vi "convertidor de pasos a distancia v1.vi"(9 "Set 0 vitual":bool, 10 "Respuesta Zaber":T7 {"Command" items=["Constant Speed Tracking"=8, "Echo"=55, "Error"=255, "Home"=1, "Limit Active"=9, "Manual Move Tracking"=10, "Move Absolute"=20, "Move at Constant Speed"=22, "Move Relative"=21, "Renumber"=2, "Restore Settings"=36, "Stop"=23]}, 11 "Datos adquisición Input":T1={"Equipo a Utilizar"=enum."TDS 2012B Osciloscope", "Montura"=enum."Motor Bipolar", "Datos Zaber"={"Sentido de Adquisición"=FALSE, "Comenzar Desde Home?"=FALSE, "Distancia a recorrer (um)"=0.0, "Pasos motor"=0, "Distancia entre Lecturas (um)"=0.0, "Puerto"=""}, "Datos Bipolar/Unipolar"={"Puerto COM"="", "Pasos entre Lecturas"=0, "Numero de lecturas"=0, "Sentido del motor"=TRUE}, "Datos Archivo"={"Ruta Archivo"=path "", "Nombre de Prueba"=""}, "Datos actuales"={"Montura"="", "Equipo"="", "Posición Actual"="", "Distancia Total a recorrer"="", "distancia Entre lecturas"="", "Pasos entre lecturas"=""}, "Datos a Guardar In"={"Datos Cursor Tektronix"="", "Datos Lokin"="", "Posición Cero"=0.0, "Posición Actual"=0.0}, "Datos Osciloscopio"={"Sesión Visa Osciloscopio"="Tektronix_TDS2012C", "Tipo de Adquisición"=enum."Voltaje Pico Pico", "Canal a Utilizar"=enum."Canal 1", "Parametros de Adquisición"=enum."Una Muestra", "Número Promedio"=2}, "Datos Lock In"={"Visa Lock in"="Tektronix_TDS2012C"}} {"Datos Osciloscopio"."Número Promedio" min=2 max=20; "Datos a Guardar In"."Posición Actual" format="%#_10f"; "Datos a Guardar In"."Posición Cero" format="%#_10f"; "Datos Bipolar/Unipolar"."Numero de lecturas" max=910098 step=1}) -> (1 "Respuesta conversión zaber":dbl[unit], 3 "Datos adquisición Out":T1={"Equipo a Utilizar"=enum."TDS 2012B Osciloscope", "Montura"=enum."Motor Bipolar", "Datos Zaber"={"Sentido de Adquisición"=FALSE, "Comenzar Desde Home?"=FALSE, "Distancia a recorrer (um)"=0.0, "Pasos motor"=0, "Distancia entre Lecturas (um)"=0.0, "Puerto"=""}, "Datos Bipolar/Unipolar"={"Puerto COM"="", "Pasos entre Lecturas"=0, "Numero de lecturas"=0, "Sentido del motor"=TRUE}, "Datos Archivo"={"Ruta Archivo"=path "", "Nombre de Prueba"=""}, "Datos actuales"={"Montura"="", "Equipo"="", "Posición Actual"="", "Distancia Total a recorrer"="", "distancia Entre lecturas"="", "Pasos entre lecturas"=""}, "Datos a Guardar In"={"Datos Cursor Tektronix"="", "Datos Lokin"="", "Posición Cero"=0.0, "Posición Actual"=0.0}, "Datos Osciloscopio"={"Sesión Visa Osciloscopio"="Tektronix_TDS2012C", "Tipo de Adquisición"=enum."Voltaje Pico Pico", "Canal a Utilizar"=enum."Canal 1", "Parametros de Adquisición"=enum."Una Muestra", "Número Promedio"=2}, "Datos Lock In"={"Visa Lock in"="Tektronix_TDS2012C"}} {"Datos Osciloscopio"."Número Promedio" min=2 max=20; "Datos a Guardar In"."Posición Actual" format="%#_10f"; "Datos a Guardar In"."Posición Cero" format="%#_10f"; "Datos Bipolar/Unipolar"."Numero de lecturas" max=910098 step=1}, 5 "Seguir Moviendo":bool)   [LabVIEW 2020]
doc: "Este Vi convierte el dato recibido de el driver zaber a distancia actual en unidades de distancia"
uses:
  <instrlib>/ZaberTSeries/Public/Utility/Response.ctl
  <instrlib>/ZaberTSeries/ZaberTSeries.lvlib
  Type Definitions/Asistente de adquisicion Cluster.ctl
  Type Definitions/Datos a Guardar.ctl
  Type Definitions/datos osciloscopio.ctl
  Type Definitions/Datos Zaber.ctl
  Type Definitions/parametros motores.ctl
  H:/Mi unidad/Departamento de Ingenieria/Investigadores/Gabriel Ramos/Proyecto Monturas v13/LV Source/Type Definitions/Tipos de montura.ctl
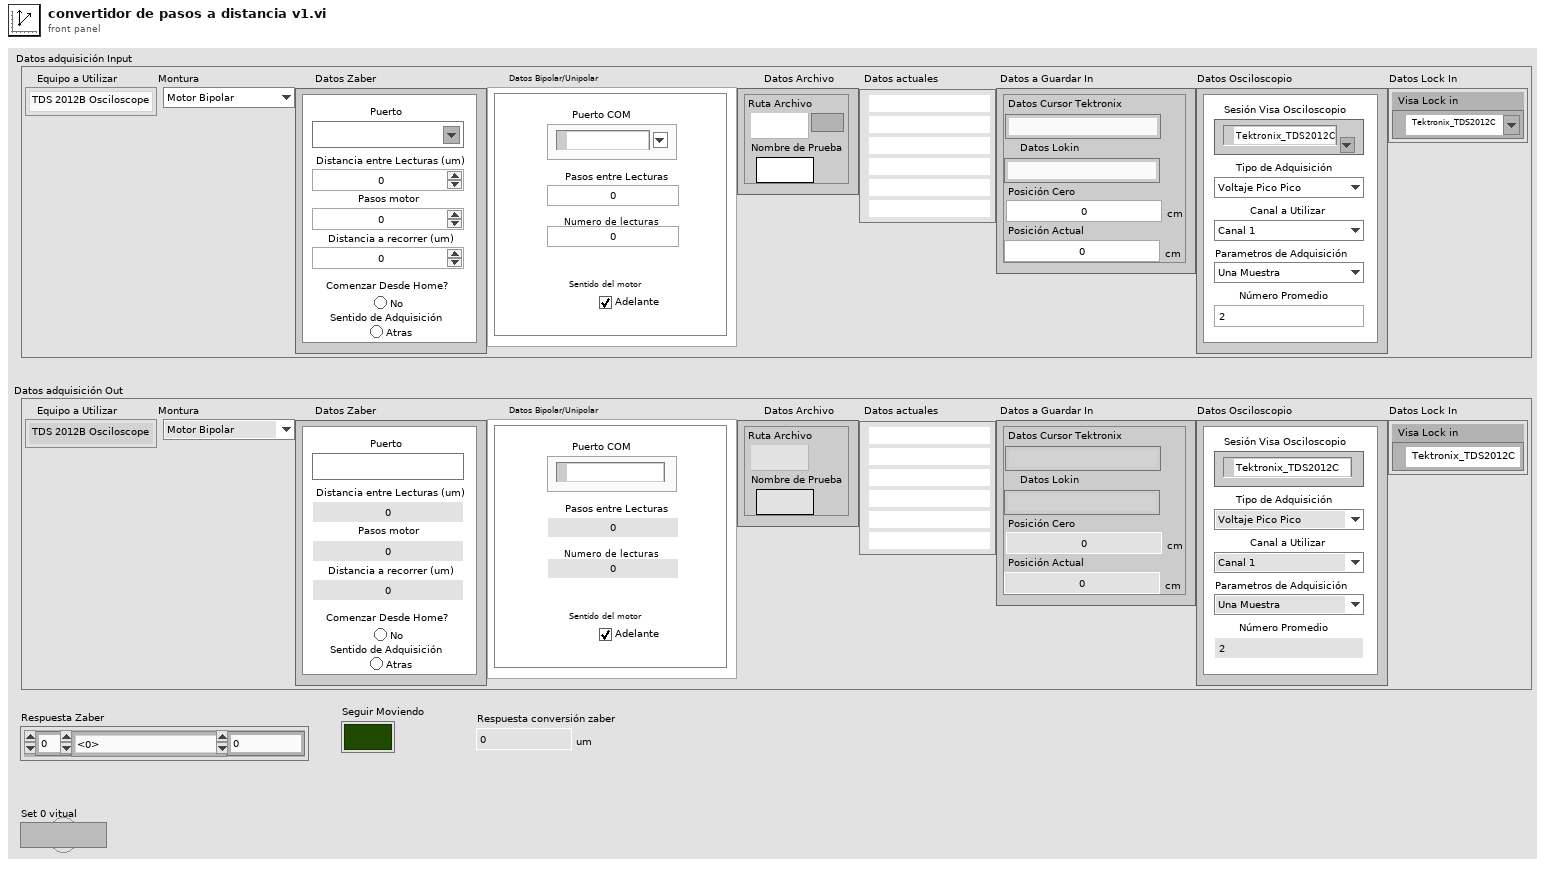
[diagram p1: front panel]
types:
  T1 = typedef "Asistente de adquisicion Cluster.ctl" = cluster{"Equipo a Utilizar":enum16{"SR830 Lock In", "TDS 2012B Osciloscope"}, "Montura":T2, "Datos Zaber":T3, "Datos Bipolar/Unipolar":T4, "Datos Archivo":cluster{"Ruta Archivo":path, "Nombre de Prueba":string}, "Datos actuales":cluster{"Montura":string, "Equipo":string, "Posición Actual":string, "Distancia Total a recorrer":string, "distancia Entre lecturas":string, "Pasos entre lecturas":string}, "Datos a Guardar In":T5, "Datos Osciloscopio":T6, "Datos Lock In":cluster{"Visa Lock in":refnum<visa-resource-name>}}
  T2 = typedef "Tipos de montura.ctl" = enum16{"Zaber T-LSR450B", "Zaber-T-LSR300B", "Zaber-T-LSRxxx", "Motor Bipolar", "Motor Unipolar"}
  T3 = typedef "Datos Zaber.ctl" = cluster{"Sentido de Adquisición":bool, "Comenzar Desde Home?":bool, "Distancia a recorrer (um)":dbl, "Pasos motor":i32, "Distancia entre Lecturas (um)":dbl, "Puerto":refnum<visa-resource-name>}
  T4 = typedef "parametros motores.ctl" = cluster{"Puerto COM":refnum<visa-resource-name>, "Pasos entre Lecturas":u16, "Numero de lecturas":u32, "Sentido del motor":bool}
  T5 = typedef "Datos a Guardar.ctl" = cluster{"Datos Cursor Tektronix":string, "Datos Lokin":string, "Posición Cero":dbl[unit], "Posición Actual":dbl[unit]}
  T6 = typedef "datos osciloscopio.ctl" = cluster{"Sesión Visa Osciloscopio":refnum<visa-resource-name>, "Tipo de Adquisición":enum16{"Voltaje Pico Pico", "Voltaje RMS", "Cursor Tiempo"}, "Canal a Utilizar":enum16{"Canal 1", "Canal 2", "Canal 1 y 2"}, "Parametros de Adquisición":enum16{"Una Muestra", "Promedio"}, "Número Promedio":i32}
  T7 = typedef "ZaberTSeries.lvlib/Response.ctl" = cluster{"Device Number":u8, "Command":u8, "Data":i32}
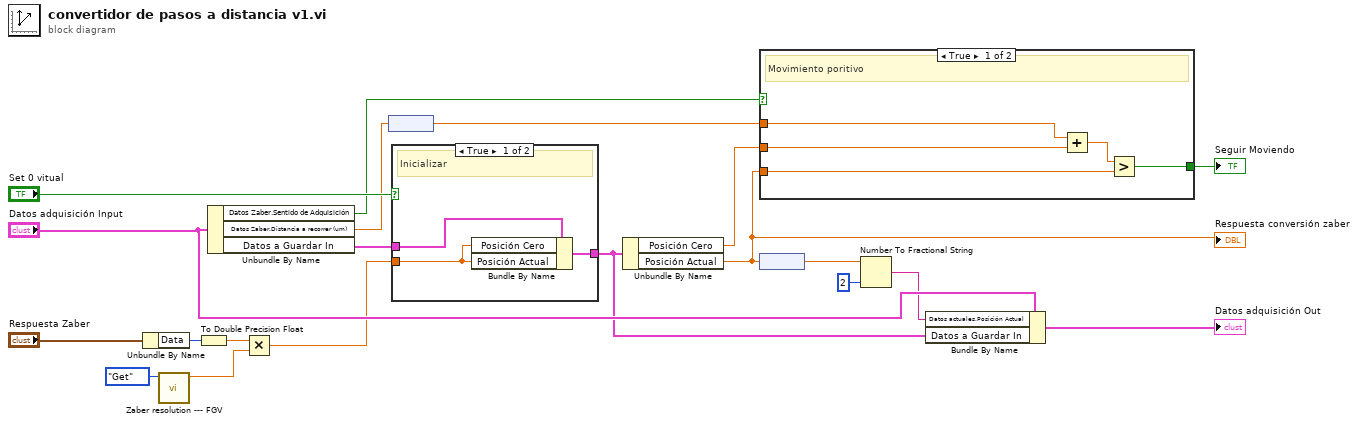
[diagram p0: block diagram]
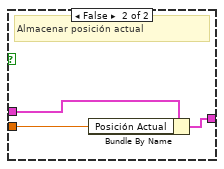
[diagram p2: hidden frame]
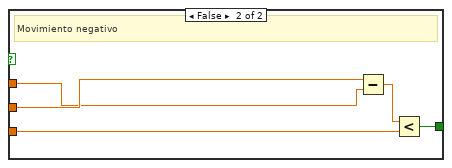
[diagram p3: hidden frame]
diagram:
  n1 = Unbundle By Name("Respuesta Zaber") -> ("Data"=w15:i32)
  n2 = call "Zaber resolution --- FGV.vi"("Action"=enum16{"Get", "Set"}."Get") -> ("Resolución"=w5:dbl[unit])  [unwired: 10 in]
  n3 = To Double Precision Float(number=w15) -> (double precision float=w4:dbl)
  n4 = Unbundle By Name("Datos adquisición Input") -> ("Datos Zaber.Sentido de Adquisición"=w16:bool, "Datos Zaber.Distancia a recorrer (um)"=w6:dbl, "Datos a Guardar In"=w12:T5)
  n5 = Multiply(x=w4, y=w5) -> (x*y=w8:dbl[unit])
  n6 = node(w6) -> (w20:dbl[unit])
  n7 = case shown="True" "Set 0 vitual" {
    tunnel: [w23 w26] -> w10
    tunnel: w12 -> [w22 w25]
    tunnel: w8 -> [w21 w24]
    frame True {
      # "Inicializar"
      n8 = Bundle By Name(cluster=w22, "Posición Cero"=w21, "Posición Actual"=w21) -> (w23:T5)
    }
    frame False {
      # "Almacenar posición actual"
      n9 = Bundle By Name(cluster=w25, "Posición Actual"=w24) -> (w26:T5)
    }
  }
  n10 = Unbundle By Name(w10) -> ("Posición Cero"=w9:dbl[unit], "Posición Actual"=w2:dbl[unit])
  "Respuesta conversión zaber" <- w2
  n11 = case shown="True" w16 {
    tunnel: w2 -> [w27 w32]
    tunnel: w20 -> [w28 w33]
    tunnel: w9 -> [w31 w34]
    tunnel: [w29 w35] -> w19
    frame True {
      # "Movimiento poritivo"
      n12 = Add(x=w28, y=w31) -> (x+y=w30:dbl[unit])
      n13 = Greater?(x=w30, y=w27) -> (0:w29:bool)
    }
    frame False {
      # "Movimiento negativo"
      n14 = Subtract(x=w34, y=w33) -> (x-y=w36:dbl[unit])
      n15 = Less?(x=w36, y=w32) -> (x < y?=w35:bool)
    }
  }
  "Seguir Moviendo" <- w19
  n16 = node(w2) -> (w3:dbl)
  n17 = Number To Fractional String(number=w3, precision (6)=i16 2) -> (F-format string=w13:string)  [unwired: 2 in]
  n18 = Bundle By Name(cluster="Datos adquisición Input", "Datos actuales.Posición Actual"=w13, "Datos a Guardar In"=w10) -> (→"Datos adquisición Out":T1)
